vi "NI USB GPIB Command.vi"(4 "Error In":errorcluster, 5 "Wait for instrument to respond (s)":dbl, 6 "String to Send":string="C0", 7 "VISA resource name":refnum<visa-resource-name>="GPIB1::25::INSTR") -> (0 "Error Out":errorcluster={"status"=TRUE, "code"=-1073807339, "source"="VISA Read in NI USB GPIB Command.vi"}, 1 "Return String from Device (Not all commands return a String)":string="C\r", 2 "Number of Bytes Recieved at Serial Port":u32, 3 "VISA resource name out":refnum<visa-resource-name>)   [LabVIEW 2016, in "IPS-120.lvlib"]
uses:
  IPS-120.lvlib
panel:
  out "return count":u32
  out "Number of Bytes sent":u32=4
  # "NI Example Serial Code"
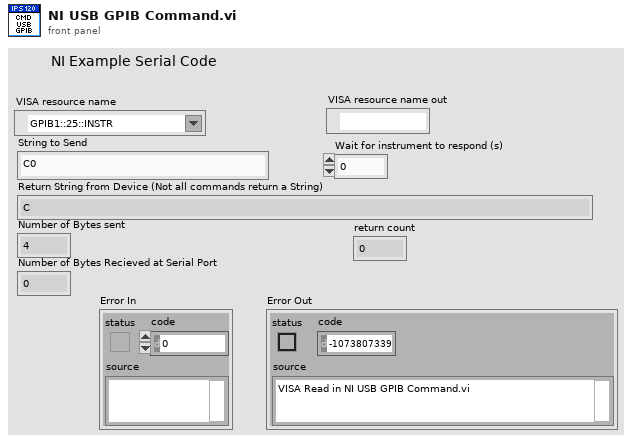
[diagram p1: front panel]
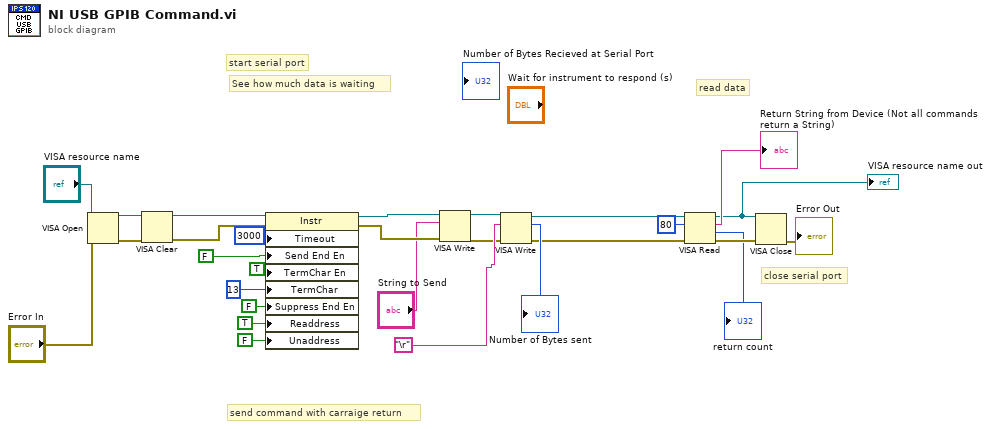
[diagram p0: block diagram]
diagram:
  # "close serial port"
  # "read data"
  # "See how much data is waiting"
  # "send command with carraige return"
  # "start serial port"
  n1 = VISA Open(error in (no error)="Error In", VISA resource name="VISA resource name") -> (VISA resource name=w14:refnum<visa-resource-name>, error out=w15:errorcluster)  [unwired: 3 in]
  n2 = VISA Clear(VISA resource name=w14, error in (no error)=w15) -> (VISA resource name out=w12:refnum<visa-resource-name>, error out=w13:errorcluster)
  n3 = property class="Instr"(reference=w12, error in=w13, "Timeout"=u32 3000 ("General Settings:Timeout Value"), "Send End En"=FALSE ("Message Based Settings:Send End Enable"), "TermChar En"=TRUE ("Message Based Settings:Termination Character Enable"), "TermChar"=u8 13 ("Message Based Settings:Termination Character"), "Suppress End En"=FALSE ("Message Based Settings:Suppress End Enable"), "Readdress"=TRUE ("GPIB Settings:Readdressing"), "Unaddress"=FALSE ("GPIB Settings:Unaddressing")) -> (reference out=w10:refnum<visa-resource-name>, error out=w11:errorcluster)
  n4 = VISA Write(VISA resource name=w10, write buffer="String to Send", error in (no error)=w11) -> (VISA resource name out=w6:refnum<visa-resource-name>, error out=w7:errorcluster)  [unwired: 1 out]
  n5 = VISA Write(VISA resource name=w6, write buffer="\r", error in (no error)=w7) -> (VISA resource name out=w25:refnum<visa-resource-name>, return count=→"Number of Bytes sent":u32, error out=w23:errorcluster)
  n6 = VISA Read(VISA resource name=w25, byte count=u32 80, error in (no error)=w23) -> (VISA resource name out=w1:refnum<visa-resource-name>, read buffer=→"Return String from Device (Not all commands return a String)":string, return count=→"return count":u32, error out=w28:errorcluster)
  "VISA resource name out" <- w1
  n7 = VISA Close(VISA resource name=w1, error in (no error)=w28) -> (error out=→"Error Out":errorcluster)
